vi "流程固件设置对话框.vi"() -> ()   [LabVIEW 2016]
uses:
  <vilib>/Utility/miscctls.llb/LVPointTypeDef.ctl
panel:
  in  "修改序列号":bool
  in  "缺试剂设置":bool
  in  "校准设置":bool
  in  "关闭":bool
  in  "参数设置":bool
  in  "固件升级":bool
  in  "流程写入":bool
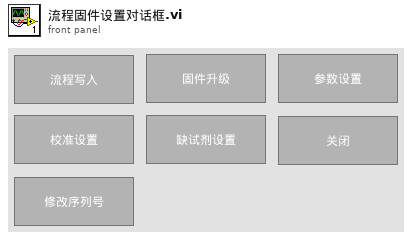
[diagram p1: front panel]
types:
  T1 = typedef "LVPointTypeDef.ctl" = cluster{"Horizontal":i16, "Vertical":i16}
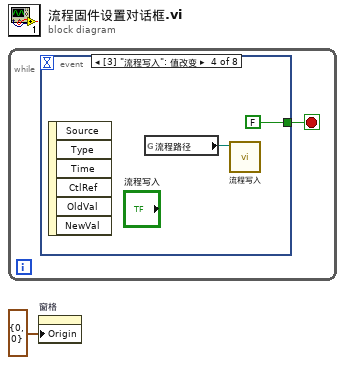
[diagram p0: block diagram]
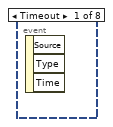
[diagram p2: hidden frame]
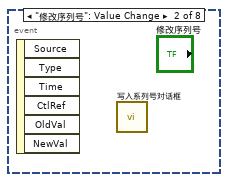
[diagram p3: hidden frame]
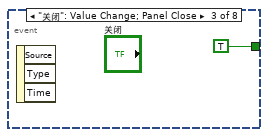
[diagram p4: hidden frame]
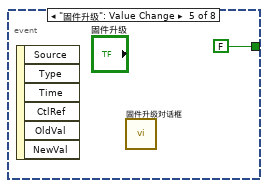
[diagram p5: hidden frame]
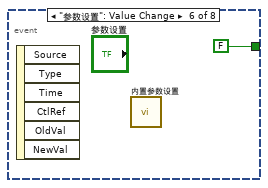
[diagram p6: hidden frame]
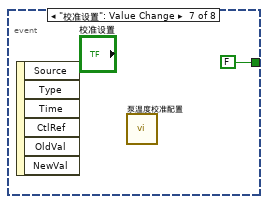
[diagram p7: hidden frame]
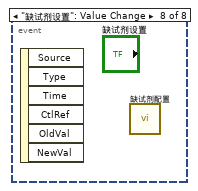
[diagram p8: hidden frame]
diagram:
  n1 = while {
    stop <- w2 stop-if-true
    n2 = event shown="[3] \"流程写入\": 值改变" {
      selector: _ -> [_ _ _ _ _ _ _ _]
      dyn-events: _ -> [_ _ _ _ _ _ _ _]
      timeout: _ -> [_ _ _ _ _ _ _ _]
      tunnel: [_ _ TRUE FALSE FALSE FALSE FALSE _] -> w2
      event Timeout {
        n3 = event-data() -> ()  [unwired: 1 in, 3 out]
      }
      event "修改序列号": Value Change {
        n4 = event-data() -> ()  [unwired: 1 in, 6 out]
        n5 = call "写入系列号对话框.vi"() -> ()  [unwired: 12 in]
      }
      event "关闭": Value Change; Panel Close {
        n6 = event-data() -> ()  [unwired: 1 in, 3 out]
      }
      event "流程写入": Value Change {
        n7 = event-data() -> ()  [unwired: 1 in, 6 out]
        n8 = global read "挥发酚断电保存全局变量.vi" "流程路径"() -> (w4:path)
        n9 = call "流程写入.vi"("添加的路径"=w4) -> ()  [unwired: 11 in]
      }
      event "固件升级": Value Change {
        n10 = event-data() -> ()  [unwired: 1 in, 6 out]
        n11 = call "固件升级对话框.vi"() -> ()  [unwired: 12 in]
      }
      event "参数设置": Value Change {
        n12 = event-data() -> ()  [unwired: 1 in, 6 out]
        n13 = call "内置参数设置.vi"() -> ()  [unwired: 12 in]
      }
      event "校准设置": Value Change {
        n14 = event-data() -> ()  [unwired: 1 in, 6 out]
        n15 = call "泵温度校准配置.vi"() -> ()  [unwired: 12 in]
      }
      event "缺试剂设置": Value Change {
        n16 = event-data() -> ()  [unwired: 1 in, 6 out]
        n17 = call "缺试剂配置.vi"() -> ()  [unwired: 12 in]
      }
    }
  }
  n18 = property on="窗格" class="Pane"("Origin"=T1 {"Horizontal"=0, "Vertical"=0} ("原点")) -> ()  [unwired: 2 in, 2 out]
